vi "Tell Parent Forward.vi"(7 "Actor in":refnum<class "Actor.lvclass">, 8 "Error in":errorcluster, 10 "Msg Attributes":refnum<data-value>) -> (0 "Error out":errorcluster, 5 "Actor out":refnum<class "Actor.lvclass">)   [LabVIEW 2020, in "_Template.lvlib" / "Templates.lvlib" / "TEMPLATE jettl Msg.lvlib" / "TEMPLATE.lvlib"]
uses:
  TEMPLATE.lvlib
  TEMPLATE jettl Msg.lvlib
  jettl/jettl/jettl.lvlib
  jettl/jettl/Actor/Actor.lvclass
  jettl/jettl/Relation.ctl
  jettl/jettl/Teller.ctl
  jettl/jettl/Msg Input/Msg Input.lvclass
  jettl/jettl/Msg Output/Msg Output.lvclass
  jettl/jettl/Msg/Msg.lvclass
  jettl/jettl/Msg Attributes.ctl
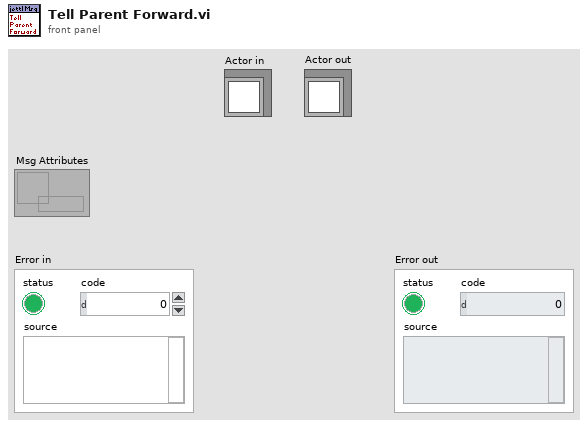
[diagram p1: front panel]
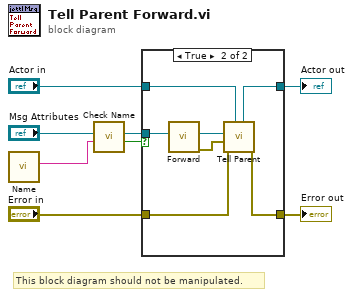
[diagram p0: block diagram]
diagram:
  # "This block diagram should not be manipulated."
  n1 = call "Name.vi"() -> ("Name"=w4:string)  [unwired: 11 in]
  n2 = call "Check Name.vi"("Name"=w4, "Msg Attributes in"="Msg Attributes") -> ("Match"=w1:bool, "Msg Attributes out"=w2:refnum<data-value>)  [unwired: 7 in, 1 out]
  n3 = case shown="True" w1 {
    tunnel: "Error in" -> [w9 w16]
    tunnel: "Actor in" -> [w10 w15]
    tunnel: [w9 w13] -> w6
    tunnel: [w10 w12] -> w5
    tunnel: w2 -> [_ w11]
    frame False {
    }
    frame True {
      n4 = call "Forward.vi"("Msg Attributes in"=w11) -> ("Error out"=w14:errorcluster, "Msg Attributes out"=w17:refnum<data-value>)  [unwired: 9 in]
      n5 = call "Tell Parent.vi"("Actor in"=w15, "Error in"=w16, "Error"=w14, "Msg Attributes"=w17) -> ("Error out"=w13:errorcluster, "Actor out"=w12:refnum<class "Actor.lvclass">)  [unwired: 6 in]
    }
  }
  "Error out" <- w6
  "Actor out" <- w5
